vi "dead band filter.vi"(7 "deadband":dbl, 11 "input":dbl) -> (3 "output":dbl)   [LabVIEW 2023]
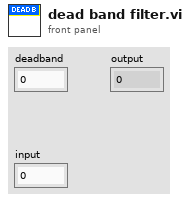
[diagram p1: front panel]
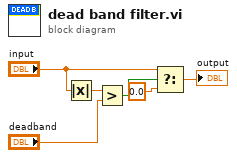
[diagram p0: block diagram]
diagram:
  n1 = Absolute Value(x="input") -> (abs(x)=w1:dbl)
  n2 = Greater?(x=w1, y="deadband") -> (0:w3:bool)
  n3 = Select(t="input", s=w3, f=0.0) -> (s? t:f=→"output":dbl)
